vi "1B Spoof Wind Acceleartation.vi"(1 "Perceived Wind":cluster{"X Position":dbl, "Y Position":dbl}, 2 "Old Velocity":dbl[](array[numeric])) -> (0 "New Velocity":dbl[](array[numeric]))   [LabVIEW 2011]
uses:
  <vilib>/Analysis/_algsub.llb/Real Vector Norm.vi
  <vilib>/Analysis/baseanly.llb/Real Dot Product.vi
  <vilib>/Analysis/NI_AALPro.lvlib
  <vilib>/Analysis/NI_AALBase.lvlib
panel:
  out "Ratio":dbl
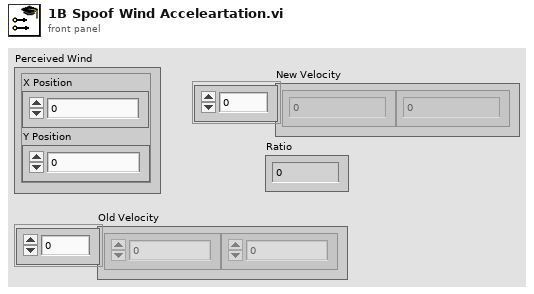
[diagram p1: front panel]
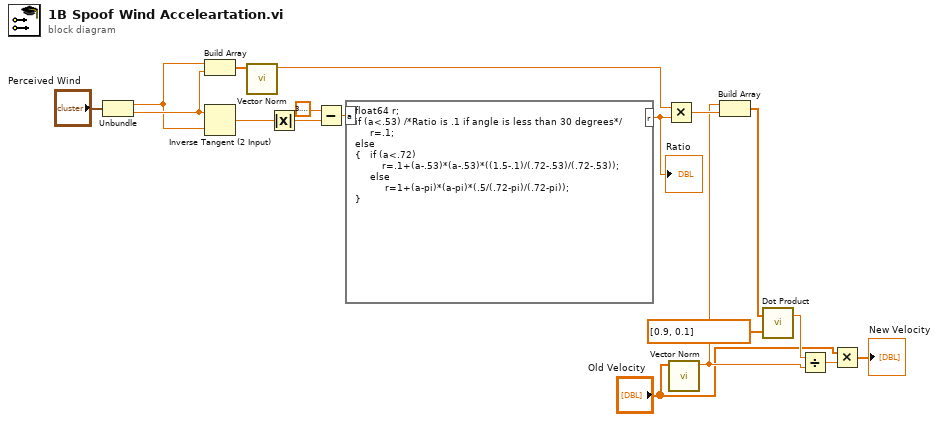
[diagram p0: block diagram]
diagram:
  n1 = Unbundle("Perceived Wind") -> ("X Position"=w1:dbl, "Y Position"=w2:dbl)
  n2 = Build Array(w1, w2) -> (w11:dbl[])
  n3 = Inverse Tangent (2 Input)(1:w1, 2:w2) -> (0:w10:dbl)
  n4 = call-poly <vilib>:"Vector Norm.vi"("Input Vector"=w11) -> ("norm"=w12:dbl)  [unwired: 9 in, 1 out]
  n5 = Absolute Value(x=w10) -> (abs(x)=w4:dbl)
  n6 = Subtract(x=3.141592653589793, y=w4) -> (x-y=w3:dbl)
  n7 = formula code="float64 r;\nif (a<.53) /*Ratio is .1 if angle is less than 30 degrees*/\n     r=.1;\nelse\n{   if (a<.72)\n         r=.1+(a-.53)*(a-.53)*((1.5-.1)/(.72-.53)/(.72-.53));\n     else\n          r=1+(a-pi)*(a-pi)*(.5/(.72-pi)/(.72-pi));\n}"("a"=w3) -> ("r"=w13:dbl)
  "Ratio" <- w13
  n8 = Multiply(x=w12, y=w13) -> (x*y=w15:dbl)
  n9 = call-poly <vilib>:"Vector Norm.vi"("Input Vector"="Old Velocity") -> ("norm"=w14:dbl)  [unwired: 9 in, 1 out]
  n10 = Build Array(w14, w15) -> (w16:dbl[])
  n11 = call-poly <vilib>:"Dot Product.vi"("Y Vector"=dbl[] [0.9, 0.1], "X Vector"=w16) -> ("X * Y"=w18:dbl)  [unwired: 1 out]
  n12 = Divide(x=w18, y=w14) -> (x/y=w6:dbl)
  n13 = Multiply(x="Old Velocity", y=w6) -> (x*y=→"New Velocity":dbl[])
